vi "HEWH Input Rate Flow Calculation.vi"(7 "Delta T Target":dbl, 8 "error in (no error)":errorcluster, 9 "Heating Value (BTU/ft³)":dbl, 11 "HEWH Data":T1={"HEWH Standard"={"Voltage (Volts)"=236.2, "Current (Amps)"=17.749, "Power (Watts)"=4192.0, "WattHours (Wh)"=0.0, "TC Tree (AVG)"=0.0, "Flow Rate (GPM)"=0.0, "Gallons (Gal)"=0.0, "RTD Out (Deg F)"=0.0, "RTD In (Deg F)"=0.0, "RTD Amb (Deg F)"=0.0, "TC Down"=0.0, "UE Event Lead"=0, "LE Event Lead"=0, "TC Tree Array"=[]}, "PRAT"={"Power (Watts) A"=4192.0, "Power (Watts) B"=4192.0, "Power (Watts) C"=4192.0, "Power (Watts) D"=4192.0, "TC1"=0.0, "TC2"=0.0, "TC3"=0.0, "TC4"=0.0, "WattHours (Wh) A"=4192.0, "WattHours (Wh) B"=4192.0, "WattHours (Wh) C"=4192.0, "WattHours (Wh) D"=4192.0, "Ambient"=0.0, "Extra Temp"=0.0}, "Additional Power Data"={"Vthd"=236.2, "Frequency (Hz)"=236.2, "Apparent Power (VA)"=236.2, "Power Factor"=236.2, "Current Crest Factor"=236.2, "Voltage Crest Factor"=236.2, "Integration Time (sec)"=236.2}}) -> (0 "error out":errorcluster, 3 "Target Flow Rate (GPM)":dbl)   [LabVIEW 2016]
uses:
  Type Definitions/HEWH Power Data.ctl
  Utility/Type Definitions/UTILITY Notifier.ctl
panel:
  in  "RTD In (Deg F) 2":dbl
  in  "RTD Out (Deg F) 2":dbl
  out "Density (lb/gal) 2":dbl format="%#.6g"
  out "Cp Water 2":dbl
  out "Target Flow Rate (GPM) 2":dbl
  in  "Delta T Target 2":dbl
  out "Thermal Efficiency (%) 2":dbl
  out "A 2":dbl
  out "B 2":dbl
  out "Volume 2":dbl
  out "Delta T 2":dbl
  in  "error in (no error) 2":errorcluster
  out "error out 2":errorcluster
  in  "Heating Value (BTU/ft³) 2":dbl
  out "Thermal Efficiency (%)":dbl
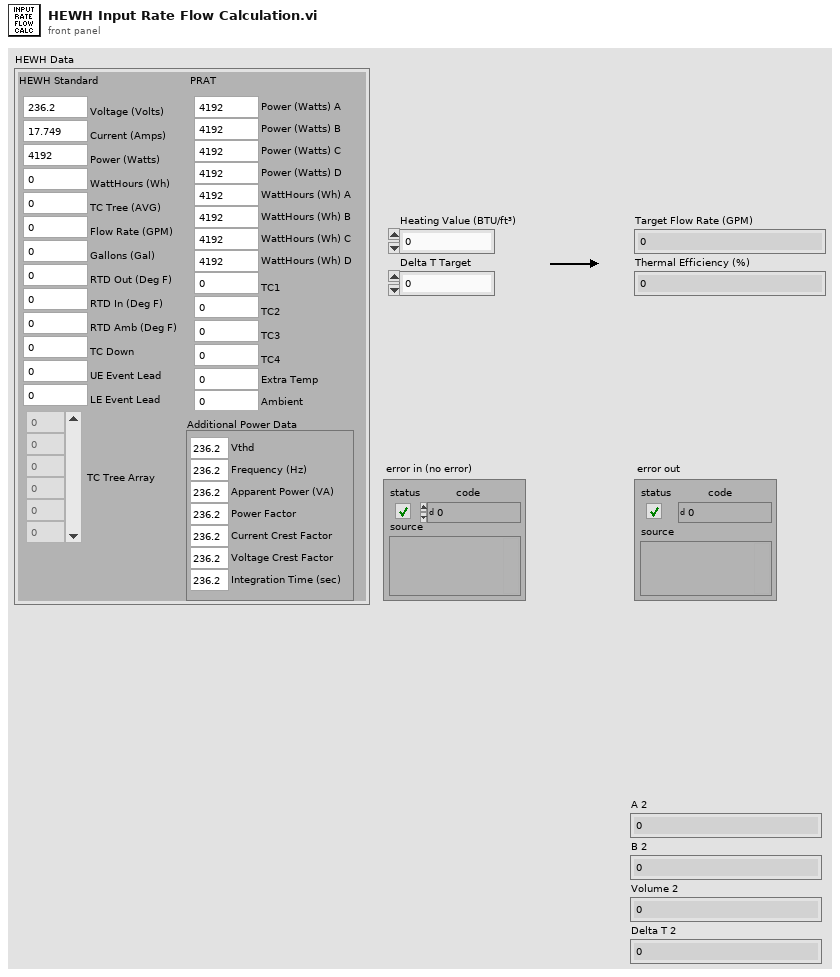
[diagram p1: front panel]
types:
  T1 = typedef "HEWH Power Data.ctl" = cluster{"HEWH Standard":cluster{"Voltage (Volts)":dbl, "Current (Amps)":dbl, "Power (Watts)":dbl, "WattHours (Wh)":dbl, "TC Tree (AVG)":dbl, "Flow Rate (GPM)":dbl, "Gallons (Gal)":dbl, "RTD Out (Deg F)":dbl, "RTD In (Deg F)":dbl, "RTD Amb (Deg F)":dbl, "TC Down":dbl, "UE Event Lead":i32, "LE Event Lead":i32, "TC Tree Array":dbl[]}, "PRAT":cluster{"Power (Watts) A":dbl, "Power (Watts) B":dbl, "Power (Watts) C":dbl, "Power (Watts) D":dbl, "TC1":dbl, "TC2":dbl, "TC3":dbl, "TC4":dbl, "WattHours (Wh) A":dbl, "WattHours (Wh) B":dbl, "WattHours (Wh) C":dbl, "WattHours (Wh) D":dbl, "Ambient":dbl, "Extra Temp":dbl}, "Additional Power Data":cluster{"Vthd":dbl, "Frequency (Hz)":dbl, "Apparent Power (VA)":dbl, "Power Factor":dbl, "Current Crest Factor":dbl, "Voltage Crest Factor":dbl, "Integration Time (sec)":dbl}}
  T2 = typedef "UTILITY Notifier.ctl" = enum16{"Set", "Read", "Release Ref"}
  T3 = typedef "Data Cluster.ctl" = cluster{"Absolute Pressure":dbl, "Gauge/Diff. Pressure":dbl, "Barometric Pressure":dbl, "Temperature":dbl, "Volumetric Flow":dbl, "Mass Flow":dbl, "Setpoint":dbl, "Valve Drive":dbl, "Totalizer":dbl, "[hr]":dbl, "[min]":dbl, "[sec]":dbl, "Totalizer Average Flow":dbl, "Totalizer Peak Flow":dbl, "Gas selected":string}
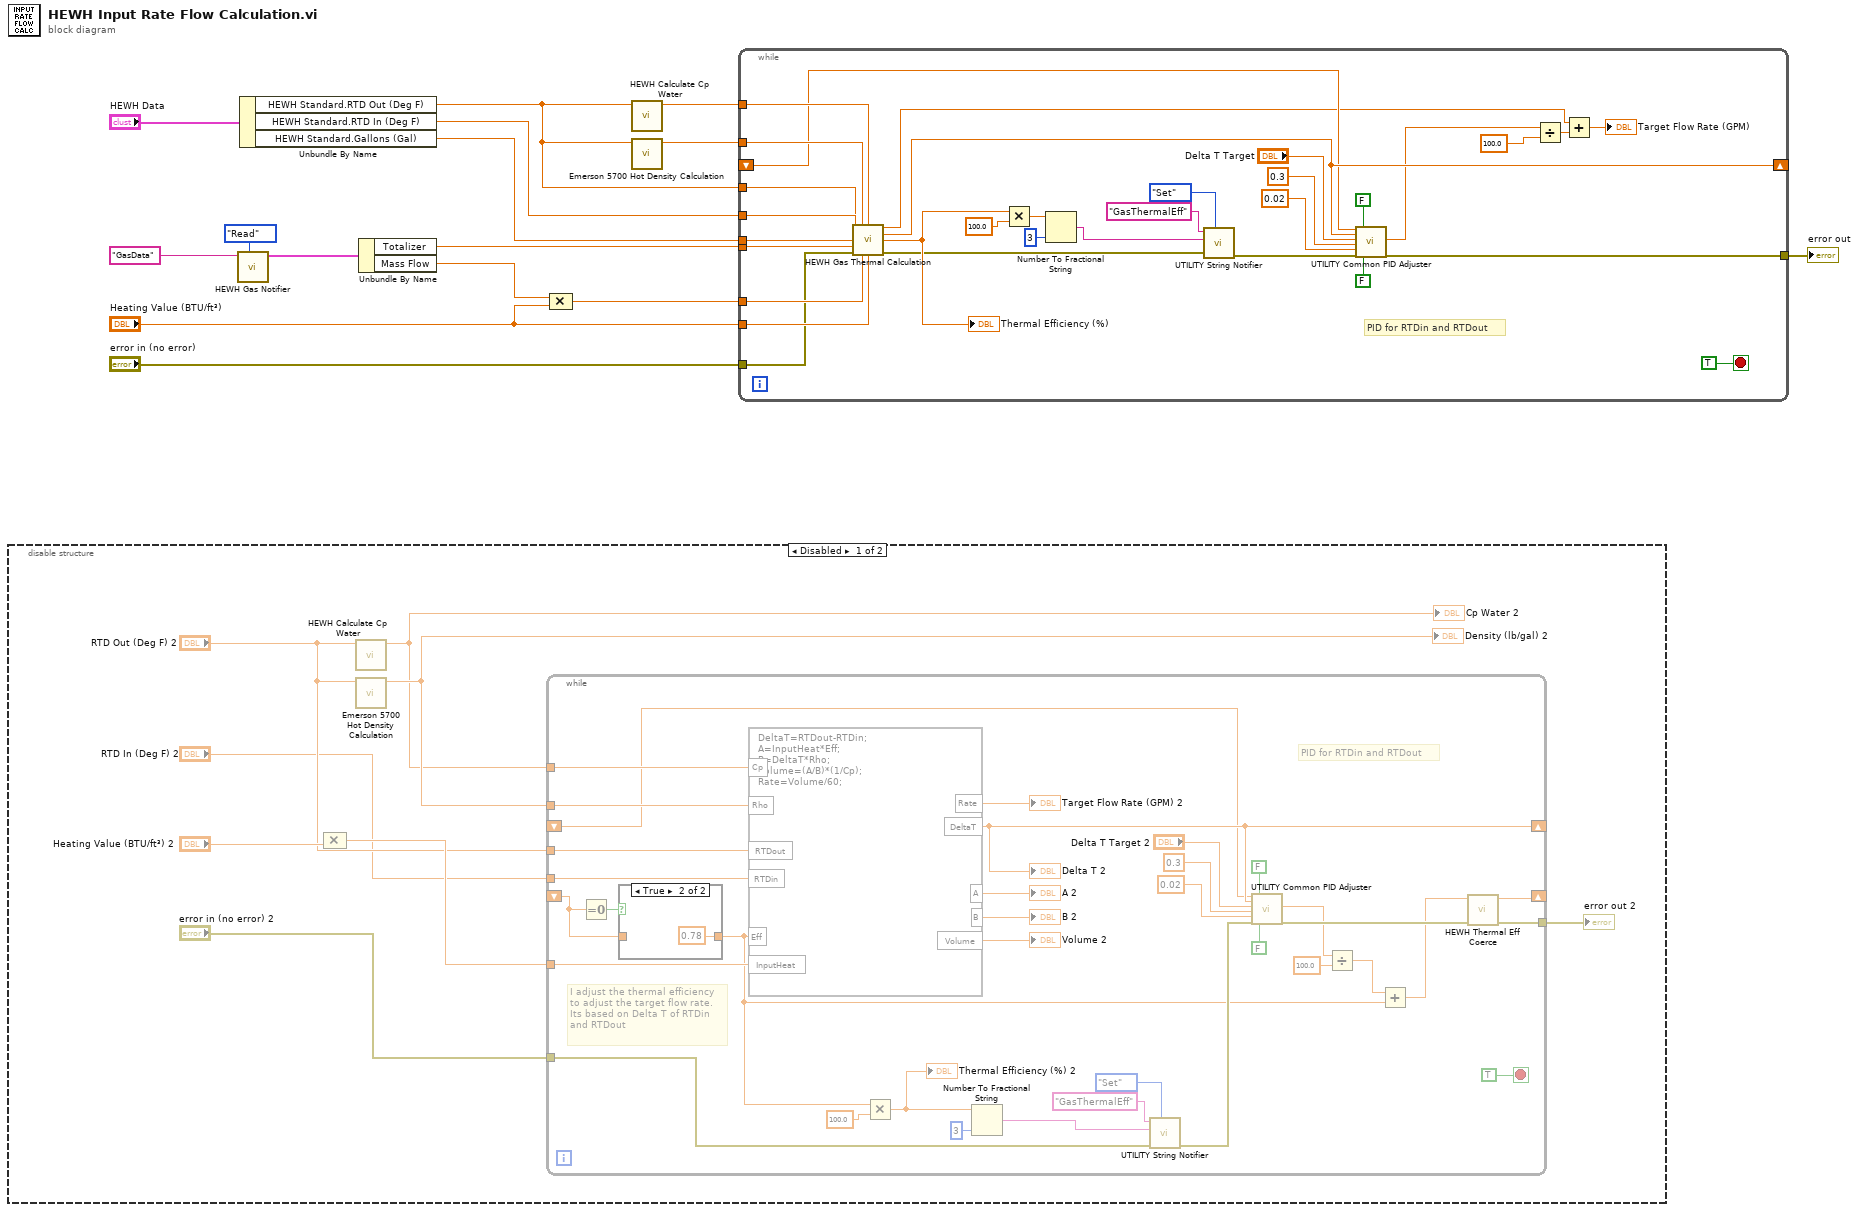
[diagram p0: block diagram]
diagram:
  n1 = disable-structure shown="Disabled" {
    frame Disabled {
      n2 = Compound Arithmetic op=MULTIPLY("Heating Value (BTU/ft³) 2") -> (w20:dbl)  [unwired: 1 in]
      n3 = call "HEWH Calculate Cp Water.vi"("RTD Out (Deg F)"="RTD Out (Deg F) 2") -> ("Cp Water"=w18:dbl)  [unwired: 10 in]
      "Cp Water 2" <- w18
      n4 = call "Emerson 5700 Hot Density Calculation.vi"("RTD Out (°F)"="RTD Out (Deg F) 2") -> ("Density (lb/gal)"=w19:dbl)  [unwired: 9 in, 1 out]
      "Density (lb/gal) 2" <- w19
      n5 = while {
        tunnel: "RTD In (Deg F) 2" -> [w58]
        tunnel: "RTD Out (Deg F) 2" -> [w57]
        tunnel: w18 -> [w55]
        tunnel: w19 -> [w54]
        tunnel: w20 -> [w53]
        shift-right: [w44] -> _
        shift-left: _ -> [w46]
        tunnel: "error in (no error) 2" -> [w32]
        tunnel: [w42] -> w22
        shift-right: [w41] -> _
        shift-left: _ -> [w40]
        stop <- TRUE stop-if-true
        # "PID for RTDin and RTDout"
        # "I adjust the thermal efficiency\nto adjust the target flow rate.\nIts based on Delta T of RTDin\nand RTDout"
        n6 = Equal To 0?(x=w46) -> (x = 0?=w47:bool)
        n7 = case shown="True" w47 {
          tunnel: [w59 0.78 ("Thermal eff (%)")] -> w29
          tunnel: w46 -> [w59 _]
          frame False {
          }
          frame True {
          }
        }
        n8 = formula code="DeltaT=RTDout-RTDin;\nA=InputHeat*Eff;\nB=DeltaT*Rho;\nVolume=(A/B)*(1/Cp);\nRate=Volume/60;"("Cp"=w55, "Rho"=w54, "RTDout"=w57, "RTDin"=w58, "Eff"=w29, "InputHeat"=w53) -> ("Rate"=→"Target Flow Rate (GPM) 2":dbl, "A"=→"A 2":dbl, "DeltaT"=w41:dbl, "B"=→"B 2":dbl, "Volume"=→"Volume 2":dbl)
        "Delta T 2" <- w41
        n9 = Multiply(x=w29, y=100.0) -> (x*y=w24:dbl)
        "Thermal Efficiency (%) 2" <- w24
        n10 = Number To Fractional String(number=w24, precision (6)=i16 3) -> (F-format string=w33:string)  [unwired: 2 in]
        n11 = call "UTILITY String Notifier.vi"("Status"=UTILITY_Notifier."Set", "error in (no error)"=w32, "Set Status"=w33, "name (unnamed)"="GasThermalEff") -> ("error out"=w31:errorcluster)  [unwired: 6 in, 1 out]
        n12 = call "UTILITY Common PID Adjuster.vi"("Previous Value"=w40, "Current Rate"=w41, "Scan Rate Target"="Delta T Target 2", "K(7) - Adjustment Factor"=0.3, "ErrorPassBand(%)"=0.02, "Error In"=w31, "Use Fuzzy Logic"=FALSE, "Use Proportion Valve"=FALSE) -> ("Adjustment Factor"=w27:dbl, "Error Out"=w43:errorcluster)  [unwired: 8 in, 2 out]
        n13 = Divide(x=w27, y=100.0) -> (x/y=w25:dbl)
        n14 = Add(x=w25, y=w29) -> (x+y=w28:dbl)
        n15 = call "HEWH Thermal Eff Coerce.vi"("error in (no error)"=w43, "Eff Input"=w28) -> ("error out"=w42:errorcluster, "Eff Output"=w44:dbl)  [unwired: 8 in]
      }
      "error out 2" <- w22
    }
    frame Enabled {
    }
  }
  n16 = call "HEWH Gas Notifier.vi"("Status"=UTILITY_Notifier."Read", "name (unnamed)"="GasData") -> ("Gas Measurment Data Output"=w1:T3)  [unwired: 8 in, 1 out]
  n17 = Unbundle By Name("HEWH Data") -> ("HEWH Standard.RTD Out (Deg F)"=w7:dbl, "HEWH Standard.RTD In (Deg F)"=w6:dbl, "HEWH Standard.Gallons (Gal)"=w5:dbl)
  n18 = Unbundle By Name(w1) -> ("Totalizer"=w9:dbl, "Mass Flow"=w12:dbl)
  n19 = Compound Arithmetic op=MULTIPLY(w12, "Heating Value (BTU/ft³)") -> (w15:dbl)
  n20 = call "HEWH Calculate Cp Water.vi"("RTD Out (Deg F)"=w7) -> ("Cp Water"=w11:dbl)  [unwired: 10 in]
  n21 = call "Emerson 5700 Hot Density Calculation.vi"("RTD Out (°F)"=w7) -> ("Density (lb/gal)"=w10:dbl)  [unwired: 9 in, 1 out]
  n22 = while {
    tunnel: w6 -> [w92]
    tunnel: w7 -> [w91]
    tunnel: w11 -> [w90]
    tunnel: w10 -> [w89]
    tunnel: w15 -> [w69]
    tunnel: "error in (no error)" -> [w63]
    tunnel: [w67] -> w13
    shift-right: [w82] -> _
    shift-left: _ -> [w81]
    tunnel: w9 -> [w72]
    tunnel: w5 -> [w74]
    tunnel: "Heating Value (BTU/ft³)" -> [w70]
    stop <- TRUE stop-if-true
    # "PID for RTDin and RTDout"
    n23 = call "HEWH Gas Thermal Calculation.vi"("RTD Out (Deg F)"=w91, "Density (lb/gal)"=w89, "Cp Water"=w90, "RTD In (Deg F)"=w92, "Gallons (Gal)"=w74, "Totalizer"=w72, "error in (no error)"=w63, "Heat Input (BTU/hr)"=w69, "Heating Value (BTU/ft³)"=w70) -> ("Target Flow Rate (GPM)"=w65:dbl, "Trise"=w82:dbl, "Eff"=w71:dbl, "error out"=w62:errorcluster)  [unwired: 3 in]
    "Thermal Efficiency (%)" <- w71
    n24 = Multiply(x=w71, y=100.0) -> (x*y=w73:dbl)
    n25 = Number To Fractional String(number=w73, precision (6)=i16 3) -> (F-format string=w76:string)  [unwired: 2 in]
    n26 = call "UTILITY String Notifier.vi"("Status"=UTILITY_Notifier."Set", "error in (no error)"=w62, "Set Status"=w76, "name (unnamed)"="GasThermalEff") -> ("error out"=w75:errorcluster)  [unwired: 6 in, 1 out]
    n27 = call "UTILITY Common PID Adjuster.vi"("Previous Value"=w81, "Current Rate"=w82, "Scan Rate Target"="Delta T Target", "K(7) - Adjustment Factor"=0.3, "ErrorPassBand(%)"=0.02, "Error In"=w75, "Use Fuzzy Logic"=FALSE, "Use Proportion Valve"=FALSE) -> ("Adjustment Factor"=w61:dbl, "Error Out"=w67:errorcluster)  [unwired: 8 in, 2 out]
    n28 = Divide(x=w61, y=100.0) -> (x/y=w66:dbl)
    n29 = Add(x=w65, y=w66) -> (x+y=→"Target Flow Rate (GPM)":dbl)
  }
  "error out" <- w13
